vi "Printer Cmnd.vi"(7 "Action?":T1, 8 "error in (no error)":errorcluster, 11 "String":string) -> (0 "error out":errorcluster, 3 "Printer Command Out":string)   [LabVIEW 2021]
uses:
  Gen fgv action.ctl
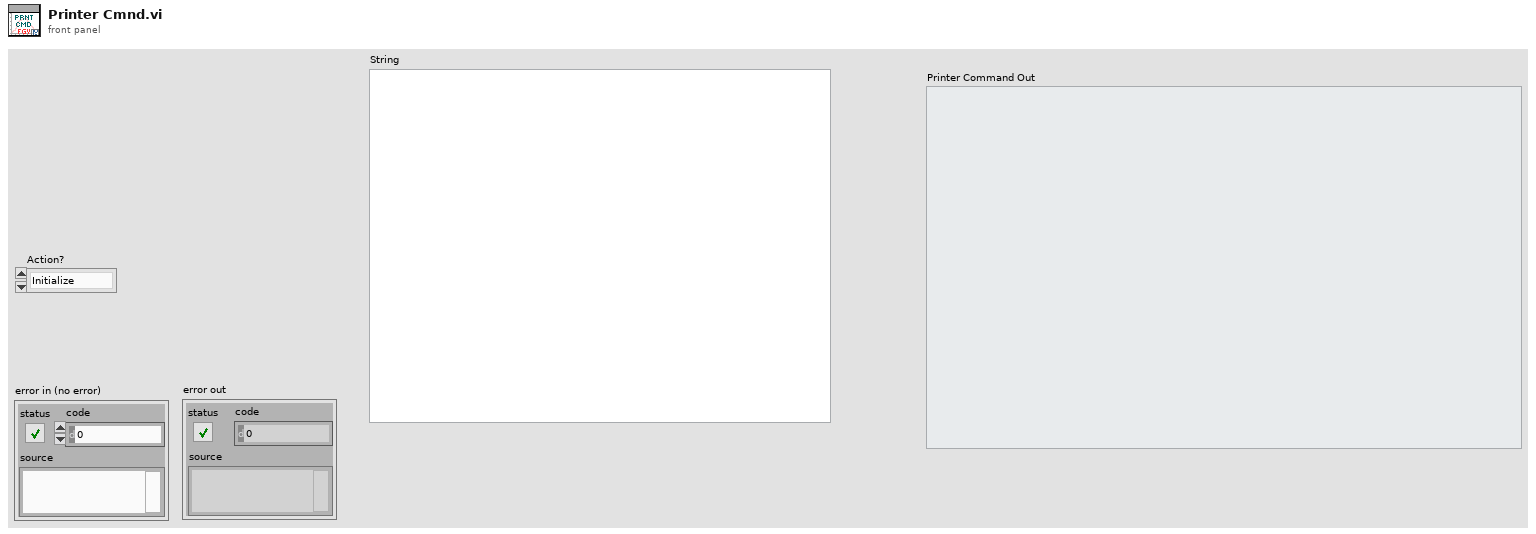
[diagram p1: front panel]
types:
  T1 = typedef "Gen FGV Action.ctl" = enum16{"Initialize", "Get Data", "Update Data", "Clear Data"}
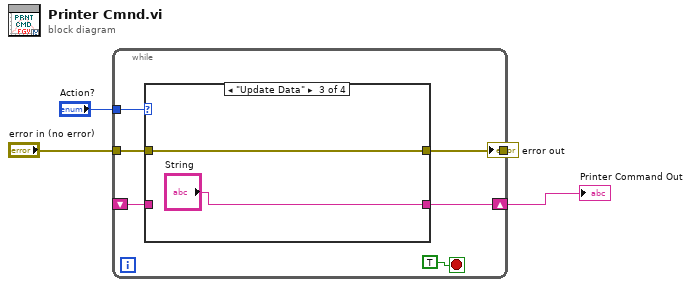
[diagram p0: block diagram]
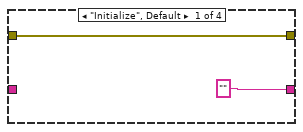
[diagram p2: hidden frame]
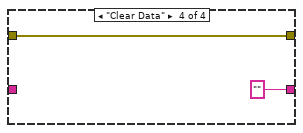
[diagram p4: hidden frame]
diagram:
  n1 = while {
    tunnel: "Action?" -> [w10]
    tunnel: [w5] -> w3
    tunnel: "error in (no error)" -> [w6]
    shift-right: [w8] -> w1
    shift-left: _ -> [w7]
    stop <- TRUE stop-if-true
    n2 = case shown="\"Update Data\"" w10 {
      tunnel: ["" w14 "String" ""] -> w8
      tunnel: w7 -> [_ w14 _ _]
      tunnel: w6 -> [w12 w13 w15 w17]
      tunnel: [w12 w13 w15 w17] -> w5
      frame "Initialize", Default {
      }
      frame "Get Data" {
      }
      frame "Update Data" {
      }
      frame "Clear Data" {
      }
    }
  }
  "error out" <- w3
  "Printer Command Out" <- w1
